vi "Set Calculation Settings.vi"(6 "Backend engine":T1, 8 "error in":errorcluster, 11 "Calculation Settings":T2={"Strict"=FALSE, "Verbose"=TRUE, "Uncertainty Calculation Method"=enum."none", "Correlations"={"Required"=FALSE, "Generate"=FALSE}, "Degrees of Freedom"={"Required"=FALSE, "Generate"=TRUE}, "MCM Calculation Settings"={"Repeats"=100, "Verbose"=TRUE, "Parallelization method"=enum."Single Core", "Processors"=1, "Temporary directory"=".", "Randomize"=TRUE}} {"MCM Calculation Settings"."Processors" min=0 step=1; "MCM Calculation Settings"."Repeats" min=1 step=1}) -> (0 "error out":errorcluster)   [LabVIEW 2013, in "QWTBLVLib.lvlib"]
doc: "Set calculation settings."
uses:
  QWTBLVLib.lvlib
  TD Calculation Settings.ctl
  TD Uncertainty Calculation Method.ctl
  TD Correlation Calculation Settings.ctl
  TD DOF Calculation Settings.ctl
  TD MCM Calculation Settings.ctl
  TD MCM Calculation Method.ctl
  TD Backend Engine.ctl
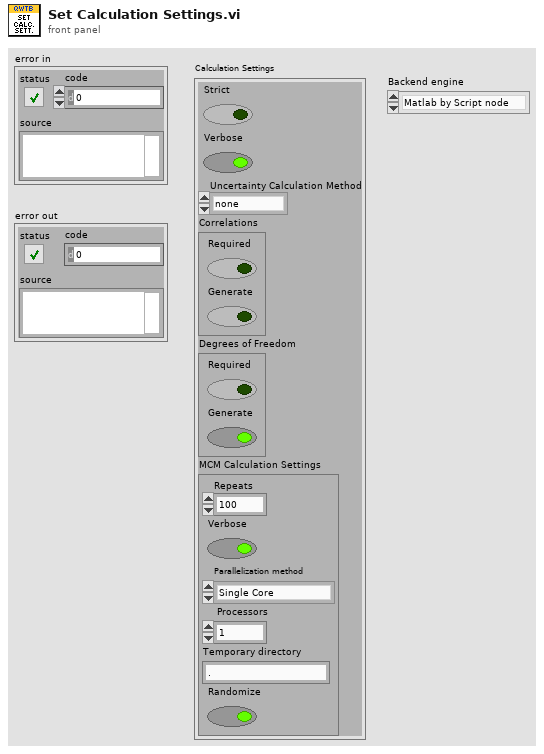
[diagram p1: front panel]
types:
  T1 = typedef "QWTBLVLib.lvlib/TD Backend Engine.ctl" = enum16{"Matlab by Script node", "GNU Octave by GOLPI"}
  T2 = typedef "QWTBLVLib.lvlib/TD Calculation Settings.ctl" = cluster{"Strict":bool, "Verbose":bool, "Uncertainty Calculation Method":T3, "Correlations":T4, "Degrees of Freedom":T5, "MCM Calculation Settings":T6}
  T3 = typedef "QWTBLVLib.lvlib/TD Uncertainty Calculation Method.ctl" = enum16{"none", "GUF", "MCM"}
  T4 = typedef "QWTBLVLib.lvlib/TD Correlation Calculation Settings.ctl" = cluster{"Required":bool, "Generate":bool}
  T5 = typedef "QWTBLVLib.lvlib/TD DOF Calculation Settings.ctl" = cluster{"Required":bool, "Generate":bool}
  T6 = typedef "QWTBLVLib.lvlib/TD MCM Calculation Settings.ctl" = cluster{"Repeats":i32, "Verbose":bool, "Parallelization method":T7, "Processors":i32, "Temporary directory":string, "Randomize":bool}
  T7 = typedef "QWTBLVLib.lvlib/TD MCM Calculation Method.ctl" = enum16{"Single Core", "Multi Core", "Multi Station"}
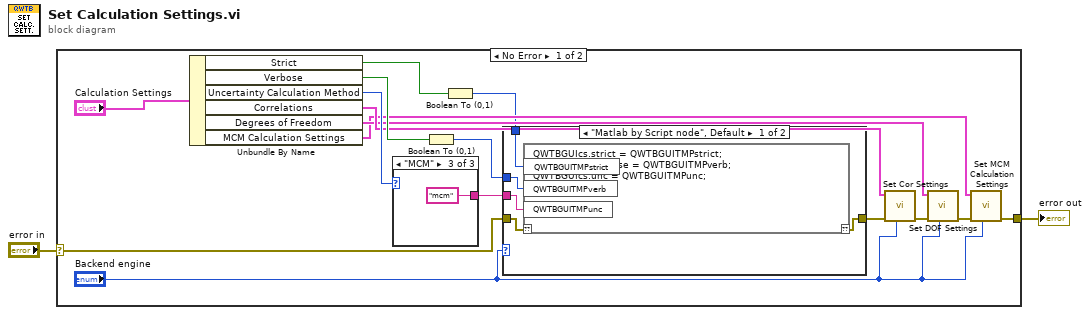
[diagram p0: block diagram]
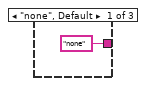
[diagram p3: hidden frame]
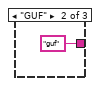
[diagram p4: hidden frame]
diagram:
  n1 = case shown="No Error" "error in" {
    selector: "error in" -> [w16 w28]
    tunnel: [w7 w28] -> w2
    frame No Error {
      n2 = Unbundle By Name("Calculation Settings") -> ("Strict"=w4:bool, "Verbose"=w13:bool, "Uncertainty Calculation Method"=w14:T3, "Correlations"=w11:T4, "Degrees of Freedom"=w9:T5, "MCM Calculation Settings"=w6:T6)
      n3 = case shown="\"MCM\"" w14 {
        tunnel: ["none" ("String") "guf" ("String") "mcm" ("String")] -> w17
        frame "none", Default {
        }
        frame "GUF" {
        }
        frame "MCM" {
        }
      }
      n4 = Boolean To (0,1)(Boolean=w13) -> (0, 1=w18:i16)
      n5 = Boolean To (0,1)(Boolean=w4) -> (0, 1=w3:i16)
      n6 = case shown="\"Matlab by Script node\", Default" "Backend engine" {
        tunnel: [w23 w24] -> w12
        tunnel: w18 -> [w22 _]
        tunnel: w17 -> [w21 _]
        tunnel: w16 -> [w20 w24]
        tunnel: w3 -> [w19 _]
        frame "Matlab by Script node", Default {
          n7 = script code="QWTBGUIcs.strict = QWTBGUITMPstrict;\nQWTBGUIcs.verbose = QWTBGUITMPverb;\nQWTBGUIcs.unc = QWTBGUITMPunc;"("??"=w20, "QWTBGUITMPverb"=w22, "QWTBGUITMPunc"=w21, "QWTBGUITMPstrict"=w19) -> ("??"=w23:errorcluster)
        }
        frame "GNU Octave by GOLPI" {
          # "#2DO"
        }
      }
      n8 = call "Set Cor Settings.vi"("Backend engine"="Backend engine", "error in"=w12, "Correlations"=w11) -> ("error out"=w10:errorcluster)  [unwired: 8 in]
      n9 = call "Set DOF Settings.vi"("Backend engine"="Backend engine", "error in"=w10, "Degrees Of Freedom"=w9) -> ("error out"=w8:errorcluster)  [unwired: 8 in]
      n10 = call "Set MCM Calculation Settings.vi"("Backend engine"="Backend engine", "error in"=w8, "MCM Calcualtion Settings"=w6) -> ("error out"=w7:errorcluster)  [unwired: 8 in]
    }
    frame Error {
    }
  }
  "error out" <- w2
